vi "DAQTriggeringTesting.vi"() -> ()   [LabVIEW 2010]
uses:
  <vilib>/DAQmx/read.llb/DAQmx Read (Analog 2D DBL NChan NSamp).vi
  <vilib>/DAQmx/create/channels.llb/DAQmx Create Channel (AI-Voltage-Basic).vi
  <vilib>/DAQmx/configure/timing.llb/DAQmx Timing (Sample Clock).vi
  <vilib>/DAQmx/configure/trigger.llb/DAQmx Reference Trigger (Digital Edge).vi
  <vilib>/daqmx/miscellaneous.llb/DAQmx Fill In Error Info.vi
panel:
  out "data":dbl[][](array[numeric]) format="%0.2f"
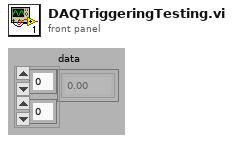
[diagram p1: front panel]
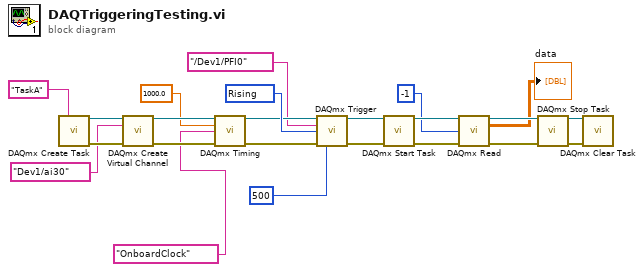
[diagram p0: block diagram]
diagram:
  w19 = 10280 items=["Rising"=10280, "Falling"=10171] ("edge")
  n1 = call <vilib>:"DAQmx Create Task.vi"("new task name"="TaskA") -> ("task out"=w21:refnum<k21>, "error out"=w20:errorcluster)  [unwired: 4 in, 9 out]
  n2 = call-poly <vilib>:"DAQmx Create Virtual Channel.vi"("task in"=w21, "physical channels"=tag "Dev1/ai30", "error in"=w20) -> ("task out"=w22:refnum<k21>, "error out"=w23:errorcluster)  [unwired: 6 in, 5 out]
  n3 = call-poly <vilib>:"DAQmx Timing.vi"("task/channels in"=w22, "rate"=1000.0, "source"=tag "OnboardClock", "error in"=w23) -> ("task out"=w18:refnum<k21>, "error out"=w17:errorcluster)  [unwired: 3 in, 7 out]
  n4 = call-poly <vilib>:"DAQmx Trigger.vi"("task/channels in"=w18, "source"=tag "/Dev1/PFI0", "edge"=w19, "error in"=w17, "pretrigger samples per channel"=u32 500) -> ("task out"=w16:refnum<k21>, "error out"=w15:errorcluster)  [unwired: 9 out]
  n5 = call <vilib>:"DAQmx Start Task.vi"("task/channels in"=w16, "error in"=w15) -> ("task out"=w12:refnum<k21>, "error out"=w11:errorcluster)  [unwired: 12 in]
  n6 = call-poly <vilib>:"DAQmx Read.vi"("task/channels in"=w12, "number of samples per channel"=-1, "error in"=w11) -> ("task out"=w6:refnum<k21>, "data"=→"data":dbl[][], "error out"=w7:errorcluster)  [unwired: 10 in]
  n7 = call <vilib>:"DAQmx Stop Task.vi"("task/channels in"=w6, "error in"=w7) -> ("task out"=w9:refnum<k21>, "error out"=w8:errorcluster)  [unwired: 12 in]
  n8 = call <vilib>:"DAQmx Clear Task.vi"("task in"=w9, "error in"=w8) -> ()  [unwired: 13 in, 1 out]
